vi "Save Copy Data.vi"(8 "error in (no error)":errorcluster, 11 "xml string":string) -> (0 "error out":errorcluster)   [LabVIEW 2021]
uses:
  <userlib>/John_Lib/TopPath/TopPath.lvlib
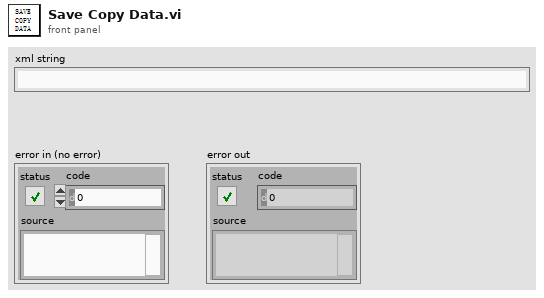
[diagram p1: front panel]
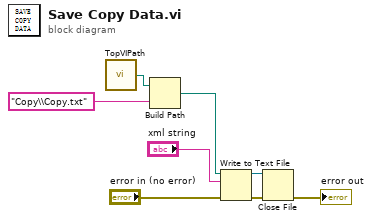
[diagram p0: block diagram]
diagram:
  n1 = call <userlib>:"TopVIPath.vi"() -> ("ConfigFile path"=w4:path)  [unwired: 2 out]
  n2 = Build Path(base path=w4, name or relative path="Copy\\Copy.txt" ("xml string")) -> (appended path=w5:path)
  n3 = Write to Text File(file (use dialog)=w5, text="xml string", error in="error in (no error)") -> (refnum out=w3:refnum<file>, error out=w2:errorcluster)  [unwired: 1 in, 1 out]
  n4 = Close File(refnum=w3, error in=w2) -> (error out=→"error out":errorcluster)  [unwired: 1 out]
